vi "ALU.vi"(0 "A":T5, 1 "Control":T4, 2 "alu_regs_flags":T2, 3 "tick":bool, 4 "clear all":bool) -> (5 "acc_content":T1, 6 "Flags":T3)   [LabVIEW 2013]
panel:
  out "b":T1
  out "a":T1
  # "0 if logical\n1 if arythmetical"
  # "R1"
  # "R1"
  # "R1"
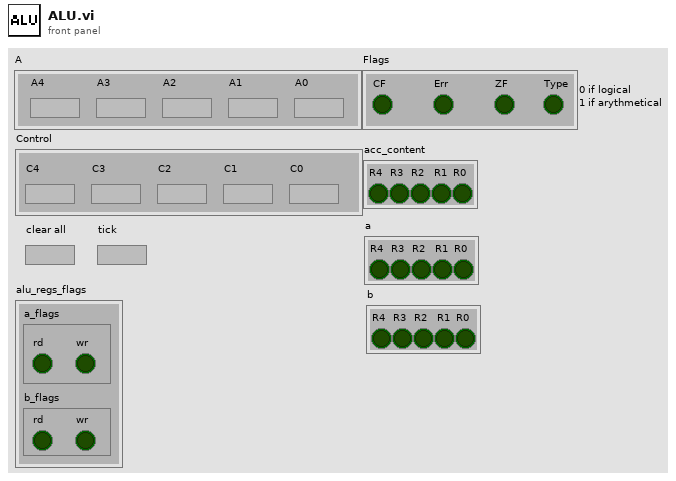
[diagram p1: front panel]
types:
  T1 = cluster{"R4":bool, "R3":bool, "R2":bool, bool, "R0":bool}
  T2 = cluster{"a_flags":cluster{"rd":bool, "wr":bool}, "b_flags":cluster{"rd":bool, "wr":bool}}
  T3 = cluster{"CF":bool, "Err":bool, "ZF":bool, "Type":bool}
  T4 = cluster{"C4":bool, "C3":bool, "C2":bool, "C1":bool, "C0":bool}
  T5 = cluster{"A4":bool, "A3":bool, "A2":bool, "A1":bool, "A0":bool}
  T6 = cluster{"Y4":bool, "Y3":bool, "Y2":bool, "Y1":bool, "Y0":bool}
  T7 = cluster{bool, "CF":bool, "Err":bool, "ZF":bool, "Type":bool}
  T8 = cluster{"Y3":bool, "Y2":bool, "Y1":bool, "Y0":bool}
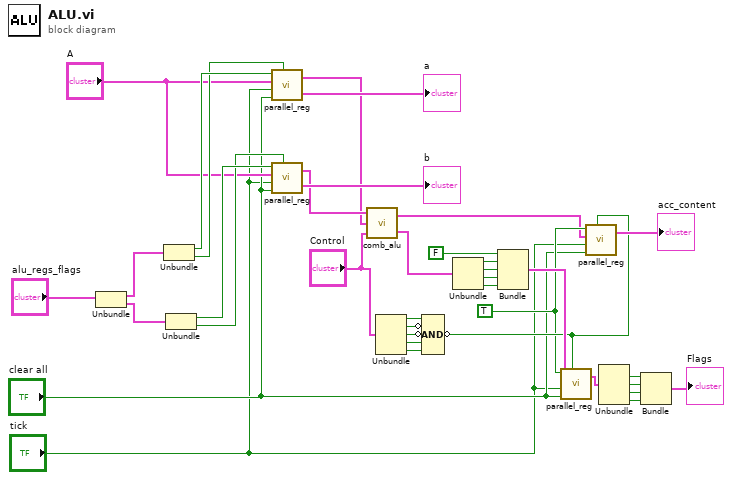
[diagram p0: block diagram]
diagram:
  w6 = TRUE
  n1 = Unbundle("alu_regs_flags") -> ("a_flags"=w22:cluster{"rd":bool, "wr":bool}, "b_flags"=w21:cluster{"rd":bool, "wr":bool})
  n2 = Unbundle(w22) -> ("rd"=w20:bool, "wr"=w19:bool)
  n3 = Unbundle(w21) -> ("rd"=w18:bool, "wr"=w17:bool)
  n4 = call "parallel_reg.vi"("RD"=w20, "I"="A", "C"="tick", "R"="clear all", "WR"=w19) -> ("O"=w1:T6, "direct_out"=→"a":T6)
  n5 = call "parallel_reg.vi"("RD"=w18, "I"="A", "C"="tick", "R"="clear all", "WR"=w17) -> ("O"=w2:T6, "direct_out"=→"b":T6)
  n6 = call "comb_alu.vi"("Control"="Control", "B"=w1, "A"=w2) -> ("Flags"=w25:T3, "Result"=w5:T1)
  n7 = Unbundle("Control") -> ("C4"=w12:bool, "C3"=w11:bool, "C2"=w10:bool, "C1"=w9:bool, "C0"=w8:bool)
  n8 = Compound Arithmetic op=AND(w12, invert w11, invert w10, w9, w8) -> (invert w7:bool)
  n9 = Unbundle(w25) -> ("CF"=w28:bool, "Err"=w29:bool, "ZF"=w30:bool, "Type"=w31:bool)
  n10 = Bundle(FALSE, "CF"=w28, "Err"=w29, "ZF"=w30, "Type"=w31) -> (w26:T7)  [unwired: 1 in]
  n11 = call "parallel_reg.vi"("RD"=w6, "I"=w26, "C"="tick", "R"="clear all", "WR"=w7) -> ("O"=w32:T6)  [unwired: 1 out]
  n12 = call "parallel_reg.vi"("RD"=w6, "I"=w5, "C"="tick", "R"="clear all", "WR"=w7) -> ("O"=→"acc_content":T6)  [unwired: 1 out]
  n13 = Unbundle(w32) -> ("Y3"=w34:bool, "Y2"=w35:bool, "Y1"=w36:bool, "Y0"=w37:bool)  [unwired: 1 out]
  n14 = Bundle("Y3"=w34, "Y2"=w35, "Y1"=w36, "Y0"=w37) -> (→"Flags":T8)  [unwired: 1 in]
